vi "readFile.vi"(8 "error in (no error)":errorcluster, 11 "Path":path=path "/home/ttsai/Documents/stash/ts_tcs_ofc/configData/pinv.esti") -> (0 "error out":errorcluster, 3 "Array":string[](array[string]))   [LabVIEW 2016]
doc: "Read the configuration file by line."
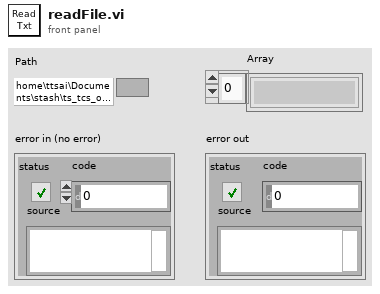
[diagram p1: front panel]
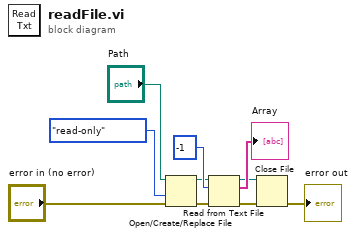
[diagram p0: block diagram]
diagram:
  n1 = Open/Create/Replace File(file path (use dialog)="Path", error in="error in (no error)", access (0:read/write)=enum16{"read/write", "read-only", "write-only"}."read-only") -> (refnum out=w4:refnum<file>, error out=w6:errorcluster)  [unwired: 3 in, 1 out]
  n2 = Read from Text File(file (use dialog)=w4, count=-1, error in=w6) -> (refnum out=w5:refnum<file>, text=→"Array":string[], error out=w7:errorcluster)  [unwired: 1 in, 1 out]
  n3 = Close File(refnum=w5, error in=w7) -> (error out=→"error out":errorcluster)  [unwired: 1 out]
